vi "SVT Power Spectrum.vi"   [LabVIEW 2017]
doc: "Computes the power spectrum of <B>scaled signal [EU]</B>. You can use this polymorphic VI to analyze signals from a single channel or from N channels. The data type you wire to the <B>scaled signal [EU]</B> input determines the polymorphic instance to use."
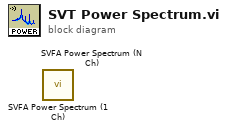
[diagram p0: block diagram]
diagram:
  n1 = call <vilib>:"SVFA Power Spectrum (1 Ch).vi"() -> ()  [unwired: 14 in, 6 out]
  n2 = call <vilib>:"SVFA Power Spectrum (N Ch).vi"() -> ()  [unwired: 14 in, 6 out]
